vi "Get Configuration Information.vi"(10 "This Application":refnum<vi>, 11 "This VI":refnum<vi>) -> (0 "error out":errorcluster, 3 "Configuration Data":T1={"Plugin Configuration Information"={"Plugin Locaiton on Disk"=path ""}, "UI Configuration Information"={"Space Between Buttons"=3, "Number of Buttons to Show"=6, "Header Image"=path "Images/Blue Background.bmp", "Footer Image"=path "Images/Blue Background.bmp"}})   [LabVIEW 2011]
uses:
  Main Type Definitions/Framework Configuration Data.ctl
  Plugin Handler/Plugin Strict Type Definitions/Plugin Configuration Information.ctl
  User Interface/UI Control Definitions/UI Configuration Information.ctl
  Root Location Global.vi
  <vilib>/Utility/config.llb/NI_LVConfig.lvlib
panel:
  in  "error in (no error)":errorcluster
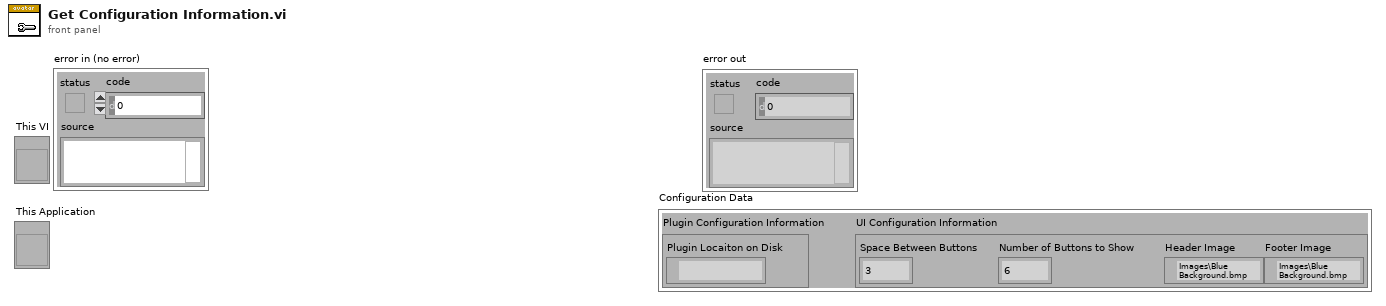
[diagram p1: front panel]
types:
  T1 = typedef "Framework Configuration Data.ctl" = cluster{"Plugin Configuration Information":T2, "UI Configuration Information":T3}
  T2 = typedef "Plugin Configuration Information.ctl" = cluster{"Plugin Locaiton on Disk":path}
  T3 = typedef "UI Configuration Information.ctl" = cluster{"Space Between Buttons":i32, "Number of Buttons to Show":i32, "Header Image":path, "Footer Image":path}
  T4 = enum32{"invalid app kind", "Development System", "Run Time System", "Student Edition", "Embedded LabVIEW", "Evaluation", "Custom"}
  T5 = typedef "NI_LVConfig.lvlib/Config Data RefNum.ctl" = refnum<k1>
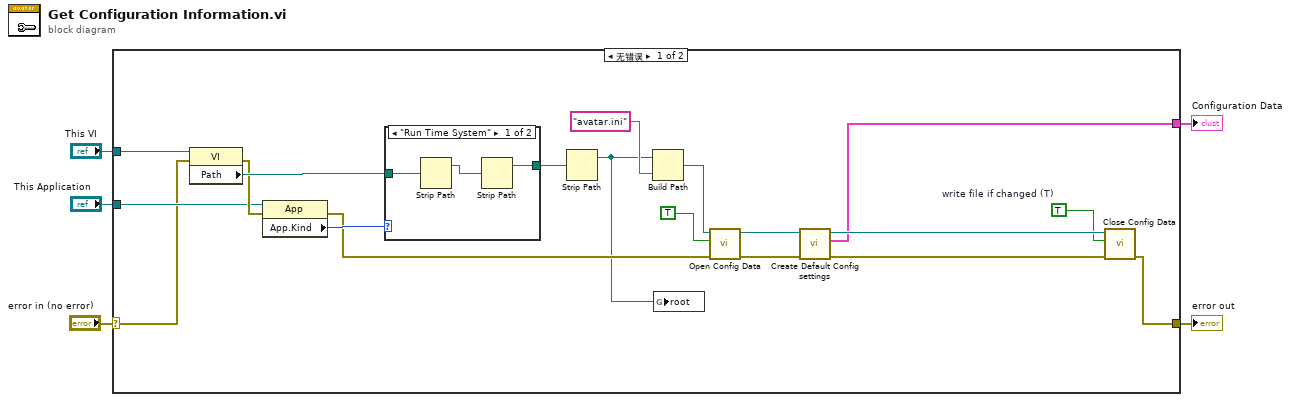
[diagram p0: block diagram]
diagram:
  n1 = case shown="无错误" "error in (no error)" {
    selector: "error in (no error)" -> [w7 w29]
    tunnel: "This Application" -> [w14 _]
    tunnel: "This VI" -> [w13 _]
    tunnel: [w11 _] -> w3
    tunnel: [w6 w29] -> w1
    frame No Error {
      w20 = TRUE  # write file if changed (T)
      n2 = property class="VI"(reference=w13, error in=w7) -> (error out=w16:errorcluster, "Path"=w17:path)  [unwired: 1 out]
      n3 = property class="App"(reference=w14, error in=w16) -> (error out=w12:errorcluster, "App.Kind"=w15:T4)  [unwired: 1 out]
      n4 = case shown="\"Run Time System\"" w15 {
        tunnel: w17 -> [w27 w28]
        tunnel: [w25 w28] -> w18
        frame "Run Time System" {
          n5 = Strip Path(path=w27) -> (stripped path=w26:path)  [unwired: 1 out]
          n6 = Strip Path(path=w26) -> (stripped path=w25:path)  [unwired: 1 out]
        }
        frame "Development System", Default {
        }
      }
      n7 = Strip Path(path=w18) -> (stripped path=w8:path)  [unwired: 1 out]
      n8 = Build Path(base path=w8, name or relative path="avatar.ini") -> (appended path=w9:path)
      n9 = global write "Root Location Global.vi" "root"(w8) -> ()
      n10 = call <vilib>:"Open Config Data.vi"("error in (no error)"=w12, "create file if necessary (T)"=TRUE, "configuration file path"=w9) -> ("error out"=w23:errorcluster, "refnum"=w21:T5)  [unwired: 6 in, 1 out]
      n11 = call "Create Default Config settings.vi"("error in"=w23, "Config File Ref"=w21) -> ("error out"=w24:errorcluster, "Configuration Data"=w11:T1, "refnum out"=w22:T5)  [unwired: 7 in]
      n12 = call <vilib>:"Close Config Data.vi"("error in (no error)"=w24, "write file if changed (T)"=w20, "refnum"=w22) -> ("error out"=w6:errorcluster)  [unwired: 7 in, 1 out]
    }
    frame Error {
    }
  }
  "error out" <- w1
  "Configuration Data" <- w3
